vi "2-4_Valves.vi"   [LabVIEW 2015]
uses:
  <vilib>/Rock Robotics/WPI/Solenoid/WPI_SolenoidChannel.ctl
  <vilib>/Rock Robotics/WPI/Solenoid/WPI_SolenoidOpenSingle.vi
  <vilib>/Rock Robotics/WPI/Utilities/WPI_GetSetVariantRefNum.vi
  Global_Var/Drive_Global.vi
  <vilib>/Rock Robotics/WPI/Solenoid/WPI_SolenoidOpenDouble.vi
panel:
  # "Created by Matt Carr on 1/25/2016"
  # "e"
types:
  T1 = typedef "WPI_SolenoidChannel.ctl" = enum8{"Solenoid 0", "Solenoid 1", "Solenoid 2", "Solenoid 3", "Solenoid 4", "Solenoid 5", "Solenoid 6", "Solenoid 7", "Invalid"}
  T2 = typedef "WPI_CompressorDevRef.ctl" = cluster{"DevStatus":errorcluster, "Pneumatics Control Module":u8}
  T3 = typedef "WPI_SolenoidDevRef.ctl" = cluster{"DevStatus":errorcluster, "Pneumatics Control Module":u8, "Forward Solenoid Channel":T1, "Reverse Solenoid Channel":T1}
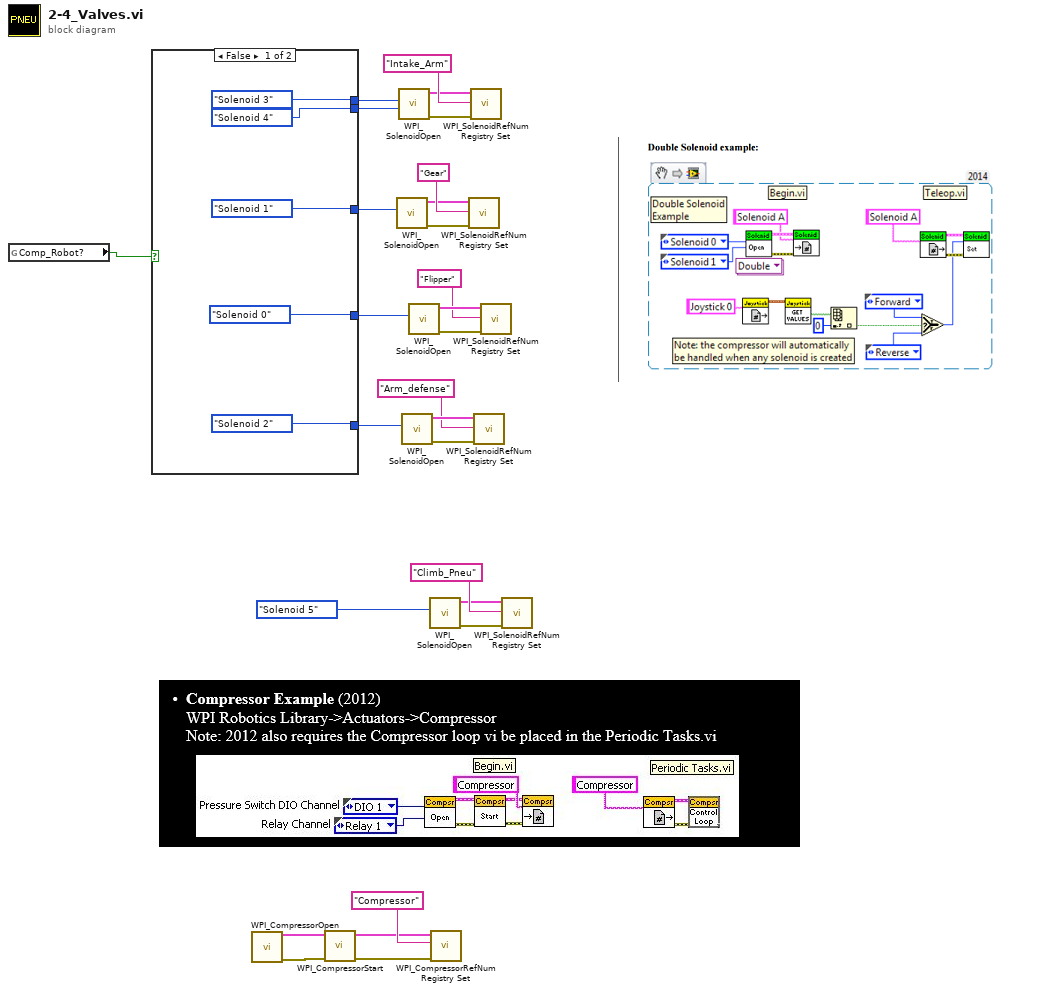
[diagram p0: block diagram]
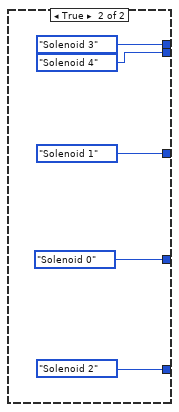
[diagram p2: hidden frame]
diagram:
  n1 = global read "Drive_Global.vi" "Comp_Robot?"() -> (w5:bool)
  n2 = case shown="False" w5 {
    tunnel: [WPI_SolenoidChannel."Solenoid 3" ("Solenoid Channel") WPI_SolenoidChannel."Solenoid 3" ("Solenoid Channel")] -> w24
    tunnel: [WPI_SolenoidChannel."Solenoid 2" ("Solenoid Channel") WPI_SolenoidChannel."Solenoid 2" ("Solenoid Channel")] -> w14
    tunnel: [WPI_SolenoidChannel."Solenoid 1" ("Forward Solenoid Channel") WPI_SolenoidChannel."Solenoid 1" ("Forward Solenoid Channel")] -> w13
    tunnel: [WPI_SolenoidChannel."Solenoid 0" ("Forward Solenoid Channel") WPI_SolenoidChannel."Solenoid 0" ("Forward Solenoid Channel")] -> w12
    tunnel: [WPI_SolenoidChannel."Solenoid 4" ("Reverse Solenoid Channel") WPI_SolenoidChannel."Solenoid 4" ("Reverse Solenoid Channel")] -> w11
    frame False {
    }
    frame True {
    }
  }
  n3 = call <vilib>:"WPI_CompressorOpen.vi"() -> ("CompressorDevRef"=w6:T2, "error out"=w9:errorcluster)  [unwired: 14 in]
  n4 = call <vilib>:"WPI_CompressorStart.vi"("error in (no error)"=w9, "CompressorDevRef"=w6) -> ("error out"=w10:errorcluster, "CompressorDevRef"=w7:T2)  [unwired: 8 in]
  n5 = call-poly <vilib>:"WPI_SolenoidOpen.vi"("Solenoid Channel"=w13) -> ("error out"=w20:errorcluster, "SolenoidDevRef"=w18:T3)  [unwired: 9 in]
  n6 = call-poly <vilib>:"WPI_SolenoidOpen.vi"("Reverse Solenoid Channel"=w11, "Forward Solenoid Channel"=w24) -> ("error out"=w23:errorcluster, "SolenoidDevRef"=w21:T3)  [unwired: 8 in]
  n7 = call-poly <vilib>:"WPI_SolenoidOpen.vi"("Solenoid Channel"=w14) -> ("error out"=w15:errorcluster, "SolenoidDevRef"=w17:T3)  [unwired: 9 in]
  n8 = call-poly <vilib>:"WPI_SolenoidOpen.vi"("Solenoid Channel"=w12) -> ("error out"=w25:errorcluster, "SolenoidDevRef"=w27:T3)  [unwired: 9 in]
  n9 = call-poly <vilib>:"WPI_SolenoidOpen.vi"("Solenoid Channel"=WPI_SolenoidChannel."Solenoid 5") -> ("error out"=w4:errorcluster, "SolenoidDevRef"=w2:T3)  [unwired: 9 in]
  n10 = call <vilib>:"WPI_CompressorRefNum Registry Set.vi"("error in (no error)"=w10, "refnum name"="Compressor", "CompressorDevRef"=w7) -> ()  [unwired: 7 in, 2 out]
  n11 = call <vilib>:"WPI_SolenoidRefNum Registry Set.vi"("error in (no error)"=w20, "refnum name"="Gear", "SolenoidDevRef"=w18) -> ()  [unwired: 7 in, 2 out]
  n12 = call <vilib>:"WPI_SolenoidRefNum Registry Set.vi"("error in (no error)"=w23, "refnum name"="Intake_Arm", "SolenoidDevRef"=w21) -> ()  [unwired: 7 in, 2 out]
  n13 = call <vilib>:"WPI_SolenoidRefNum Registry Set.vi"("error in (no error)"=w15, "refnum name"="Arm_defense", "SolenoidDevRef"=w17) -> ()  [unwired: 7 in, 2 out]
  n14 = call <vilib>:"WPI_SolenoidRefNum Registry Set.vi"("error in (no error)"=w25, "refnum name"="Flipper", "SolenoidDevRef"=w27) -> ()  [unwired: 7 in, 2 out]
  n15 = call <vilib>:"WPI_SolenoidRefNum Registry Set.vi"("error in (no error)"=w4, "refnum name"="Climb_Pneu", "SolenoidDevRef"=w2) -> ()  [unwired: 7 in, 2 out]
